vi "RealMeasure.vi"(5 "EndTime":timestamp, 7 "StartTime":timestamp, 8 "error in":errorcluster, 11 "RealMeasure":refnum<class "RealMeasure.lvclass">) -> (0 "error out":errorcluster, 3 "Passed":bool)   [LabVIEW 2020]
uses:
  ProligentResultProcessor/Measure/RealMeasure/RealMeasure.lvclass
  C:/Projects/Result Processor/src/LabVIEWResultProcessor/ProligentResultProcessor/Measure/Measure/Measure.lvclass
  ProligentResultProcessor/Measure/RealMeasureLimit/RealMeasureLimit.lvclass
  C:/Projects/Result Processor/src/LabVIEWResultProcessor/ProligentResultProcessor/Measure/RangeMeasureLimit/RangeMeasureLimit.lvclass
  C:/Projects/Result Processor/src/LabVIEWResultProcessor/ProligentResultProcessor/Measure/MeasureLimit/MeasureLimit.lvclass
  ProligentResultProcessor/Measure/RangeMeasureLimit/ComparisonType.ctl
  ProligentResultProcessor/Measure/Measure/SetStartDate.vi
  ProligentResultProcessor/Measure/Measure/SetMeasureExecutionStatus.vi
  ProligentResultProcessor/Measure/RealMeasure/SetValue.vi
  ProligentResultProcessor/Measure/RealMeasure/SetPrecision.vi
  ProligentResultProcessor/Measure/Measure/SetComments.vi
  ProligentResultProcessor/Measure/Measure/SetMeasureId.vi
  ProligentResultProcessor/Measure/Measure/GetStartDate.vi
  ProligentResultProcessor/Measure/Measure/GetMeasureExecutionStatus.vi
  ProligentResultProcessor/Measure/RealMeasure/GetValue.vi
  ProligentResultProcessor/Measure/RealMeasure/GetPrecision.vi
  ProligentResultProcessor/Measure/Measure/GetComments.vi
  ProligentResultProcessor/Measure/Measure/GetMeasureId.vi
  ProligentResultProcessor/Measure/Measure/GetLimit.vi
  ProligentResultProcessor/Measure/RealMeasureLimit/SetHigherBound.vi
  ProligentResultProcessor/Measure/RealMeasureLimit/SetLowerBound.vi
  ProligentResultProcessor/Measure/RangeMeasureLimit/GetComparisonType.vi
  ProligentResultProcessor/Measure/RealMeasureLimit/GetHigherBound.vi
  ProligentResultProcessor/Measure/RealMeasureLimit/GetLowerBound.vi
  ProligentResultProcessor/Measure/MeasureLimit/GetLimitExpression.vi
  ProligentResultProcessor/Measure/MeasureLimit/GetCustomData.vi
  ProligentResultProcessor/Measure/MeasureLimit/MeasureLimit.lvclass
  ProligentResultProcessor/Model/CustomData/CustomData.lvclass
  ProligentResultProcessor/Measure/RangeMeasureLimit/RangeMeasureLimit.lvclass
  ProligentResultProcessor/Measure/Measure/Measure.lvclass
  C:/Projects/Result Processor/src/LabVIEWResultProcessor/ProligentResultProcessor/Measure/RealMeasure/RealMeasure.lvclass
  C:/Projects/Result Processor/src/LabVIEWResultProcessor/ProligentResultProcessor/Measure/RealMeasureLimit/RealMeasureLimit.lvclass
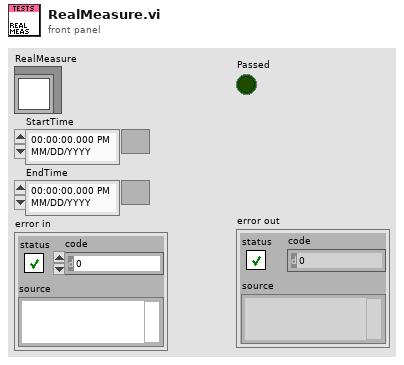
[diagram p1: front panel]
types:
  T1 = typedef "ProligentResultProcessor.lvlib/RangeMeasureLimit.lvclass/ComparisonType.ctl" = enum16{"LowerBound <= X <= HigherBound", "LowerBound < X <= HigherBound", "LowerBound <= X < HigherBound", "LowerBound < X < HigherBound", "LowerBound <= X", "LowerBound < X", "X <= HigherBound", "X < HigherBound", "X == HigherBound", "X != HigherBound", "X <= LowerBound OR HigherBound <= X", "X < LowerBound OR HigherBound <= X", "X <= LowerBound OR HigherBound < X", "X < LowerBound OR HigherBound < X"}
  T2 = enum16{"PASS", "FAIL", "NOT_COMPLETED", "ABORTED"}
  T3 = typedef "ProligentResultProcessor.lvlib/ExecutionStatus.lvclass/Value.ctl" = enum16{"PASS", "FAIL", "NOT_COMPLETED", "ABORTED"}
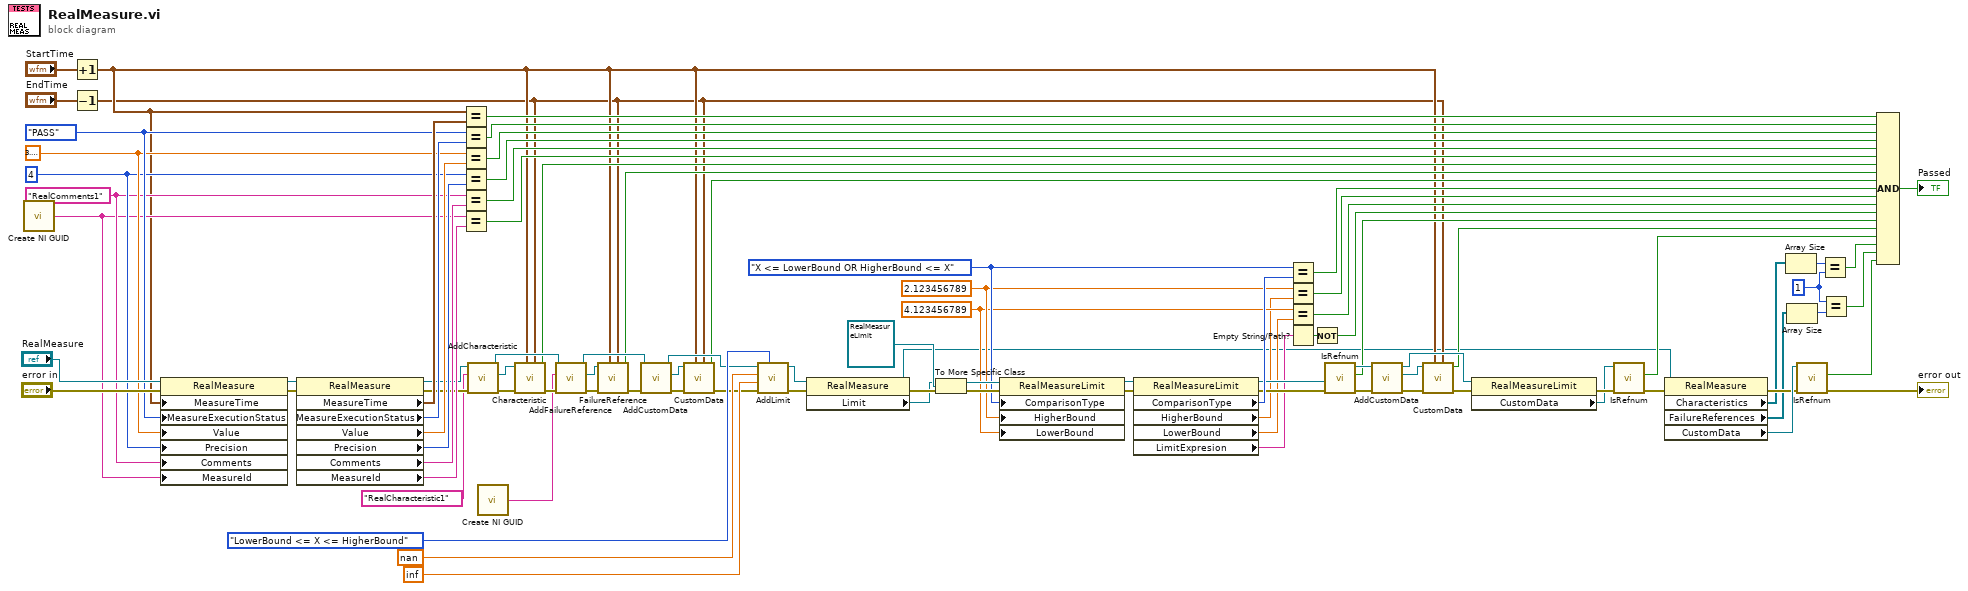
[diagram p0: block diagram]
diagram:
  w9 = 1
  w40 = "RealComments1"
  w48 = 4.123456789 ("LowerBound")
  w49 = 2.123456789 ("LowerBound")
  w50 = ComparisonType."X <= LowerBound OR HigherBound <= X" ("ComparisonType")
  w56 = u8 4
  w57 = 3.141592653589793
  w82 = T2."PASS" ("ProcessRunStatus")
  n1 = call <vilib>:"Create NI GUID.vi"() -> ("NI GUID"=w38:string)
  n2 = Increment(x="StartTime") -> (x+1=w15:timestamp)
  n3 = Decrement(x="EndTime") -> (x-1=w14:timestamp)
  n4 = property class="RealMeasure"(reference="RealMeasure", error in="error in", "MeasureTime"=w15, "MeasureExecutionStatus"=w82, "Value"=w57, "Precision"=w56, "Comments"=w40, "MeasureId"=w38) -> (reference out=w93:refnum<class "RealMeasure.lvclass">, error out=w92:errorcluster)
  n5 = property class="RealMeasure"(reference=w93, error in=w92) -> (reference out=w24:refnum<class "RealMeasure.lvclass">, error out=w21:errorcluster, "MeasureTime"=w91:timestamp, "MeasureExecutionStatus"=w90:T3, "Value"=w89:dbl, "Precision"=w55:u8, "Comments"=w39:string, "MeasureId"=w37:string)
  n6 = Equal?(x=w15, y=w91) -> (x = y?=w88:bool)
  n7 = Equal?(x=w82, y=w90) -> (x = y?=w87:bool)
  n8 = Equal?(x=w57, y=w89) -> (x = y?=w86:bool)
  n9 = Equal?(x=w56, y=w55) -> (x = y?=w45:bool)
  n10 = Equal?(x=w40, y=w39) -> (x = y?=w36:bool)
  n11 = Equal?(x=w38, y=w37) -> (x = y?=w35:bool)
  n12 = call "AddCharacteristic.vi"("error in (no error)"=w21, "FullName"="RealCharacteristic1", "Measure in"=w24) -> ("error out"=w34:errorcluster, "Characteristic"=w33:refnum<class "Characteristic.lvclass">, "Measure out"=w31:refnum<class "RealMeasure.lvclass">)  [unwired: 6 in]
  n13 = call <vilib>:"Create NI GUID.vi"() -> ("NI GUID"=w19:string)
  n14 = call "Characteristic.vi"("EndTime"=w14, "StartTime"=w15, "error in (no error)"=w34, "Characteristic in"=w33) -> ("error out"=w32:errorcluster, "Passed"=w18:bool)  [unwired: 6 in]
  n15 = call "AddFailureReference.vi"("error in (no error)"=w32, "Id"=w19, "Measure in"=w31) -> ("error out"=w26:errorcluster, "FailureReference"=w25:refnum<class "FailureReference.lvclass">, "Measure out"=w28:refnum<class "RealMeasure.lvclass">)  [unwired: 6 in]
  n16 = call "FailureReference.vi"("EndTime"=w14, "StartTime"=w15, "error in"=w26, "Defect"=w25) -> ("error out"=w30:errorcluster, "Passed"=w17:bool)  [unwired: 6 in]
  n17 = call "AddCustomData.vi"("error in (no error)"=w30, "Measure in"=w28) -> ("error out"=w29:errorcluster, "CustomData"=w27:refnum<class "CustomData.lvclass">, "Measure out"=w23:refnum<class "RealMeasure.lvclass">)  [unwired: 7 in]
  n18 = call "CustomData.vi"("EndTime"=w14, "StartTime"=w15, "error in"=w29, "CustomData"=w27) -> ("error out"=w22:errorcluster, "Passed"=w16:bool)  [unwired: 6 in]
  n19 = call "AddLimit.vi"("ComparisonType"=ComparisonType."LowerBound <= X <= HigherBound", "error in"=w22, "HigherBond"=inf ("LowerBound"), "LowerBound"=nan, "RealMeasure in"=w23) -> ("error out"=w75:errorcluster, "RealMeasure out"=w81:refnum<class "RealMeasure.lvclass">)  [unwired: 4 in, 1 out]
  n20 = property class="RealMeasure"(reference=w81, error in=w75) -> (reference out=w12:refnum<class "RealMeasure.lvclass">, error out=w80:errorcluster, "Limit"=w76:refnum<class "MeasureLimit.lvclass">)
  n21 = To More Specific Class(target class=refnum<class "RealMeasureLimit.lvclass"> refnum ("ProligentResultProcessor:RealMeasureLimit"), reference=w76, error in=w80) -> (specific class reference=w77:refnum<class "RealMeasureLimit.lvclass">, error out=w79:errorcluster)
  n22 = property class="RealMeasureLimit"(reference=w77, error in=w79, "ComparisonType"=w50, "HigherBound"=w49, "LowerBound"=w48) -> (reference out=w74:refnum<class "RealMeasureLimit.lvclass">, error out=w73:errorcluster)
  n23 = property class="RealMeasureLimit"(reference=w74, error in=w73) -> (reference out=w65:refnum<class "RealMeasureLimit.lvclass">, error out=w70:errorcluster, "ComparisonType"=w72:T1, "HigherBound"=w47:dbl, "LowerBound"=w46:dbl, "LimitExpresion"=w51:string)
  n24 = Equal?(x=w50, y=w72) -> (x = y?=w44:bool)
  n25 = Equal?(x=w49, y=w47) -> (x = y?=w43:bool)
  n26 = Equal?(x=w48, y=w46) -> (x = y?=w42:bool)
  n27 = Empty String/Path?(string/path=w51) -> (empty?=w71:bool)
  n28 = Not(x=w71) -> (.not. x?=w41:bool)
  n29 = call "IsRefnum.vi"("error in"=w70, "MeasureLimit in"=w65) -> ("error out"=w66:errorcluster, "IsRefnum"=w63:bool, "MeasureLimit out"=w64:refnum<class "RealMeasureLimit.lvclass">)  [unwired: 7 in]
  n30 = call "AddCustomData.vi"("error in"=w66, "MeasureLimit in"=w64) -> ("error out"=w61:errorcluster, "CustomData"=w59:refnum<class "CustomData.lvclass">, "MeasureLimit out"=w62:refnum<class "RealMeasureLimit.lvclass">)  [unwired: 7 in]
  n31 = call "CustomData.vi"("EndTime"=w14, "StartTime"=w15, "error in"=w61, "CustomData"=w59) -> ("error out"=w60:errorcluster, "Passed"=w58:bool)  [unwired: 6 in]
  n32 = property class="RealMeasureLimit"(reference=w62, error in=w60) -> (error out=w69:errorcluster, "CustomData"=w68:refnum<class "CustomData.lvclass">)  [unwired: 1 out]
  n33 = call "IsRefnum.vi"("error in"=w69, "CustomDataType in"=w68) -> ("error out"=w13:errorcluster, "IsRefnum"=w67:bool)  [unwired: 7 in, 1 out]
  n34 = property class="RealMeasure"(reference=w12, error in=w13) -> (error out=w6:errorcluster, "Characteristics"=w4:refnum<class "Characteristic.lvclass">[], "FailureReferences"=w3:refnum<class "FailureReference.lvclass">[], "CustomData"=w8:refnum<class "CustomData.lvclass">)  [unwired: 1 out]
  n35 = Array Size(array=w4) -> (size(s)=w11:i32)
  n36 = Array Size(array=w3) -> (size(s)=w10:i32)
  n37 = call "IsRefnum.vi"("error in"=w6, "CustomDataType in"=w8) -> ("error out"=→"error out":errorcluster, "IsRefnum"=w7:bool)  [unwired: 7 in, 1 out]
  n38 = Equal?(x=w11, y=w9) -> (x = y?=w2:bool)
  n39 = Equal?(x=w9, y=w10) -> (x = y?=w1:bool)
  n40 = Compound Arithmetic op=AND(w88, w87, w86, w45, w36, w35, w18, w17, w16, w44, w43, w42, w41, w63, w58, w67, w2, w1, w7) -> (→"Passed":bool)
